vi "dispense_on.vi"(6 "dispense status data IN":T1, 8 "error in":errorcluster, 9 "dispense run on":bool, 10 "dispense in":T2={"Vacuum Setting (0000)"=0, "Pressure"=20, "on delay (ms)"=0.5, "off delay (ms) "=0.5} {"Vacuum Setting (0000)" min=0 max=1000 step=1 format="%04.0f"}, 11 "Ultimus V2.lvclass":refnum<class "Ultimus V2.lvclass">) -> (0 "error out":errorcluster, 2 "dispense out":T2={"Vacuum Setting (0000)"=0, "Pressure"=20, "on delay (ms)"=0.5, "off delay (ms) "=0.5} {"Vacuum Setting (0000)" min=0 max=1000 step=1 format="%04.0f"}, 3 "Ultimus V2.lvclass 2":refnum<class "Ultimus V2.lvclass">, 4 "dispense status data OUT":T1)   [LabVIEW 2016]
uses:
  Classes/Controller/Dispenser/Ultimus V2 Folder/Ultimus V2.lvclass
  dispense status data.ctl
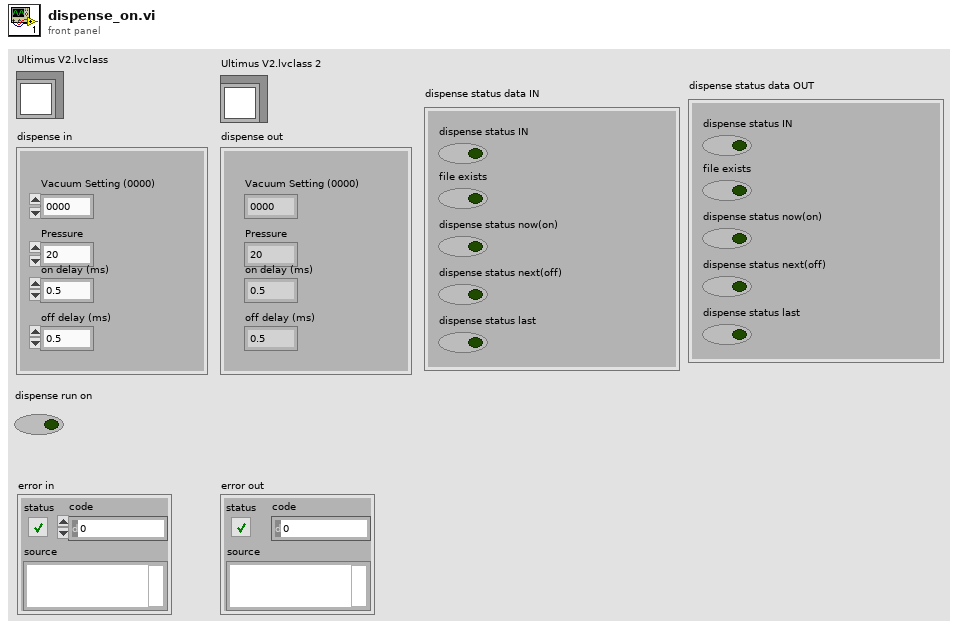
[diagram p1: front panel]
types:
  T1 = typedef "dispense status data.ctl" = cluster{"file exists":bool, "dispense status now(on)":bool, "dispense status next(off)":bool, "dispense status IN":bool, "dispense status last":bool}
  T2 = cluster{"Vacuum Setting (0000)":i64, "Pressure":i16, "on delay (ms)":dbl, "off delay (ms) ":dbl}
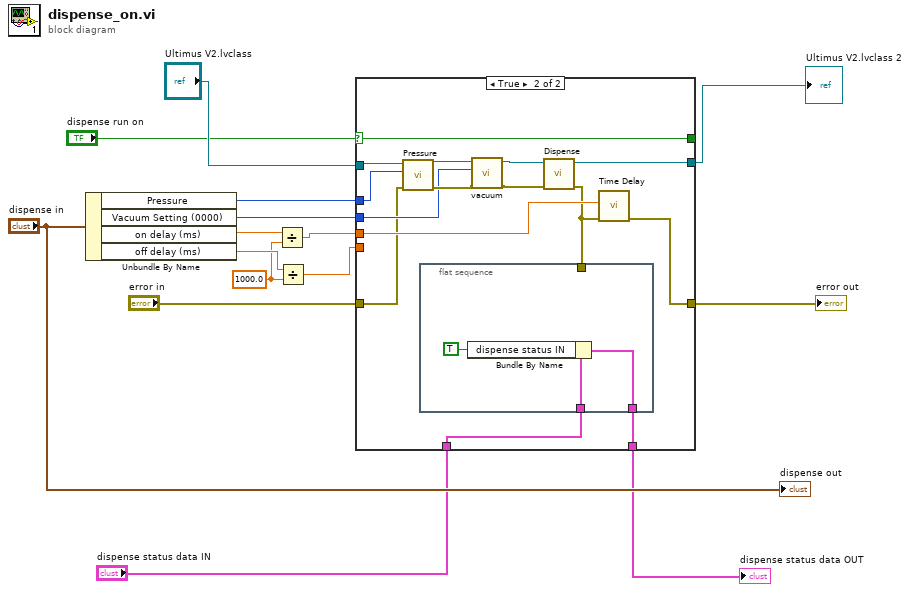
[diagram p0: block diagram]
diagram:
  w3 = 1000.0 ("y")
  n1 = Unbundle By Name("dispense in") -> ("Pressure"=w12:i16, "Vacuum Setting (0000)"=w11:i64, "on delay (ms)"=w4:dbl, "off delay (ms)"=w6:dbl)
  n2 = Divide(x=w4, y=w3) -> (x/y=w5:dbl)
  n3 = Divide(x=w6, y=w3) -> (x/y=w7:dbl)
  n4 = case shown="True" "dispense run on" {
    selector: "dispense run on" -> [w19 w23]
    tunnel: [w18 w34] -> w14
    tunnel: "Ultimus V2.lvclass" -> [w18 w32]
    tunnel: [w17 w33] -> w10
    tunnel: w11 -> [_ w27]
    tunnel: w12 -> [_ w31]
    tunnel: w5 -> [_ w25]
    tunnel: "error in" -> [w17 w24]
    tunnel: [w19 w23] -> _
    tunnel: w7 -> [_ _]
    tunnel: "dispense status data IN" -> [w16 w22]
    tunnel: [w16 w21] -> w1
    frame False {
    }
    frame True {
      n5 = call-dynamic "Pressure.vi"("error in (no error)"=w24, "Pressure"=w31, "Ultimus V in"=w32) -> ("error out"=w29:errorcluster, "Ultimus V out"=w26:refnum<class "Ultimus V2.lvclass">)  [unwired: 7 in]
      n6 = flat-sequence {
        tunnel: w22 -> [w37]
        tunnel: [w35] -> w21
        tunnel: w20 -> [_]
        frame #0 {
          n7 = Bundle By Name(cluster=w37, "dispense status IN"=TRUE) -> (w35:T1)
        }
      }
      n8 = call "vacuum.vi"("error in (no error)"=w29, "Vacuum Setting (0000)"=w27, "Ultimus V in"=w26) -> ("error out"=w28:errorcluster, "Ultimus V out"=w30:refnum<class "Ultimus V2.lvclass">)  [unwired: 7 in]
      n9 = call-dynamic "Dispense.vi"("error in (no error)"=w28, "Ultimus V in"=w30) -> ("error out"=w20:errorcluster, "Ultimus V out"=w34:refnum<class "Ultimus V2.lvclass">)  [unwired: 8 in]
      n10 = call "Time Delay"("error in (no error)"=w20, "Delay Time (s)"=w25) -> ("error out"=w33:errorcluster)  [unwired: 9 in]
    }
  }
  "Ultimus V2.lvclass 2" <- w14
  "error out" <- w10
  "dispense status data OUT" <- w1
  "dispense out" <- "dispense in"
